vi "Color Sensor V3 Match Color.vi"(11 "Measured Color":cluster{"R":dbl, "G":dbl, "B":dbl}) -> (1 "Confidence":dbl, 2 "Matched Color":cluster{"R":dbl, "G":dbl, "B":dbl}, 3 "Matched Color Name":string)   [LabVIEW 2023]
uses:
  Typedef/Color Sensor V3 FGV Command.ctl
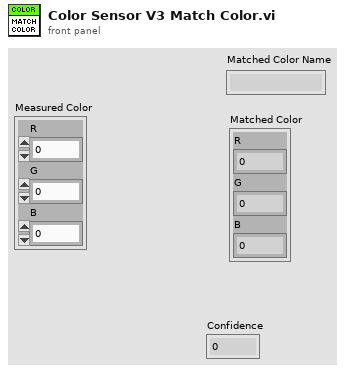
[diagram p1: front panel]
types:
  T1 = typedef "Color Sensor V3 FGV Command.ctl" = enum16{"Update", "Read"}
  T2 = typedef "Color Sensor V3 Color Match.ctl" = cluster{"Name":string, "Color":cluster{"R":dbl, "G":dbl, "B":dbl}}
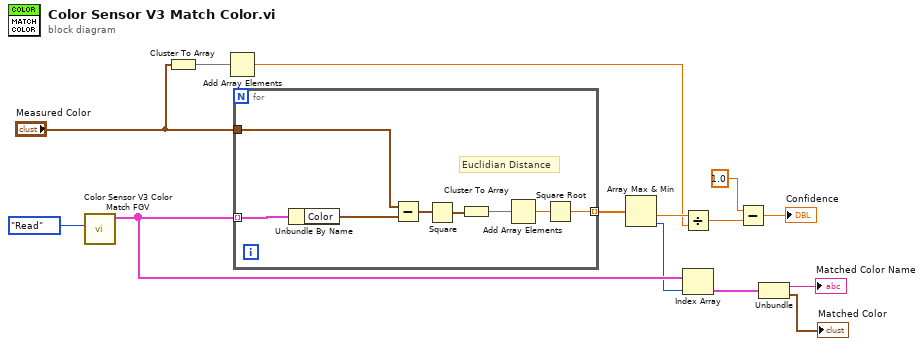
[diagram p0: block diagram]
diagram:
  n1 = call "Color Sensor V3 Color Match FGV.vi"("FGV Cmd"=Color_Sensor_V3_FGV_Command."Read" ("ColorMatchFGV-Cmd")) -> ("All Match Colors"=w11:T2[])  [unwired: 10 in]
  n2 = Cluster To Array(cluster="Measured Color") -> (array=w4:dbl[])
  n3 = Add Array Elements(numeric array=w4) -> (sum=w2:dbl)
  n4 = for {
    tunnel: w11 -> [w22] mode=indexing
    tunnel: "Measured Color" -> [w21]
    tunnel: [w15] -> w14 mode=indexing
    # "Euclidian Distance"
    n5 = Unbundle By Name(w22) -> ("Color"=w20:cluster{"R":dbl, "G":dbl, "B":dbl})
    n6 = Subtract(x=w21, y=w20) -> (x-y=w19:cluster{"R":dbl, "G":dbl, "B":dbl})
    n7 = Square(x=w19) -> (x^2=w18:cluster{"R":dbl, "G":dbl, "B":dbl})
    n8 = Cluster To Array(cluster=w18) -> (array=w17:dbl[])
    n9 = Add Array Elements(numeric array=w17) -> (sum=w16:dbl)
    n10 = Square Root(x=w16) -> (sqrt(x)=w15:dbl)
  }
  n11 = Array Max & Min(array=w14) -> (min value=w13:dbl, min index (indices)=w10:i32)  [unwired: 2 out]
  n12 = Divide(x=w13, y=w2) -> (x/y=w3:dbl)
  n13 = Index Array(array=w11, index=w10) -> (element=w9:T2)
  n14 = Subtract(x=1.0 ("max value"), y=w3) -> (x-y=→"Confidence":dbl)
  n15 = Unbundle(w9) -> ("Name"=→"Matched Color Name":string, "Color"=→"Matched Color":cluster{"R":dbl, "G":dbl, "B":dbl})
